vi "radius_plot.vi"(0 "Img Data In":T2, 11 "Controls In":T1) -> (2 "Integrated Intensity \n(Radias Direction)":i32[](graph), 4 "Img Data Out":T2, 15 "Controls Out":T1)   [LabVIEW 2023]
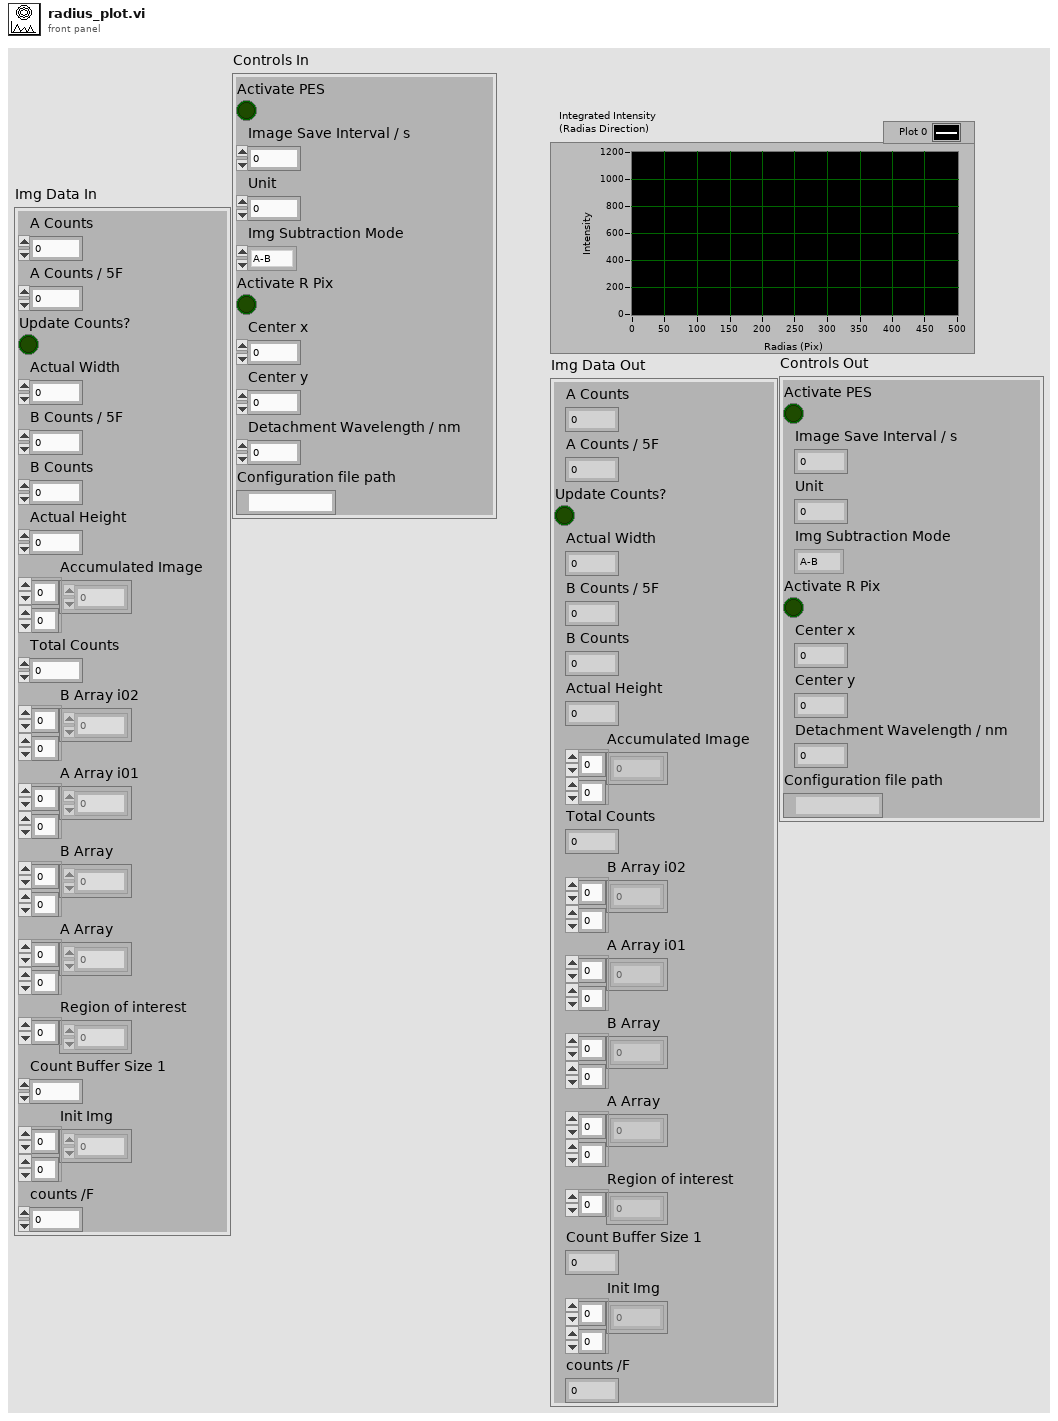
[diagram p1: front panel]
types:
  T1 = cluster{"Activate PES":bool, "Image Save Interval / s":dbl, "Unit":u16, "Img Subtraction Mode":enum16{"A-B", "B-A", "A+B"}, "Activate R Pix":bool, "Center x":i32, "Center y":i32, "Detachment Wavelength / nm":dbl, "Configuration file path":path}
  T2 = cluster{"A Counts":i32, "A Counts / 5F":dbl, "Update Counts?":bool, "Actual Width":u32, "B Counts / 5F ":dbl, "B Counts":i32, "Actual Height":u32, "Accumulated Image ":i16[][], "Total Counts":i32, "B Array i02":sgl[][], "A Array i01":sgl[][], "B Array":i16[][], "A Array":i16[][], "Region of interest":i32[], "Count Buffer Size 1":i32, "Init Img":i16[][], "counts /F":i16}
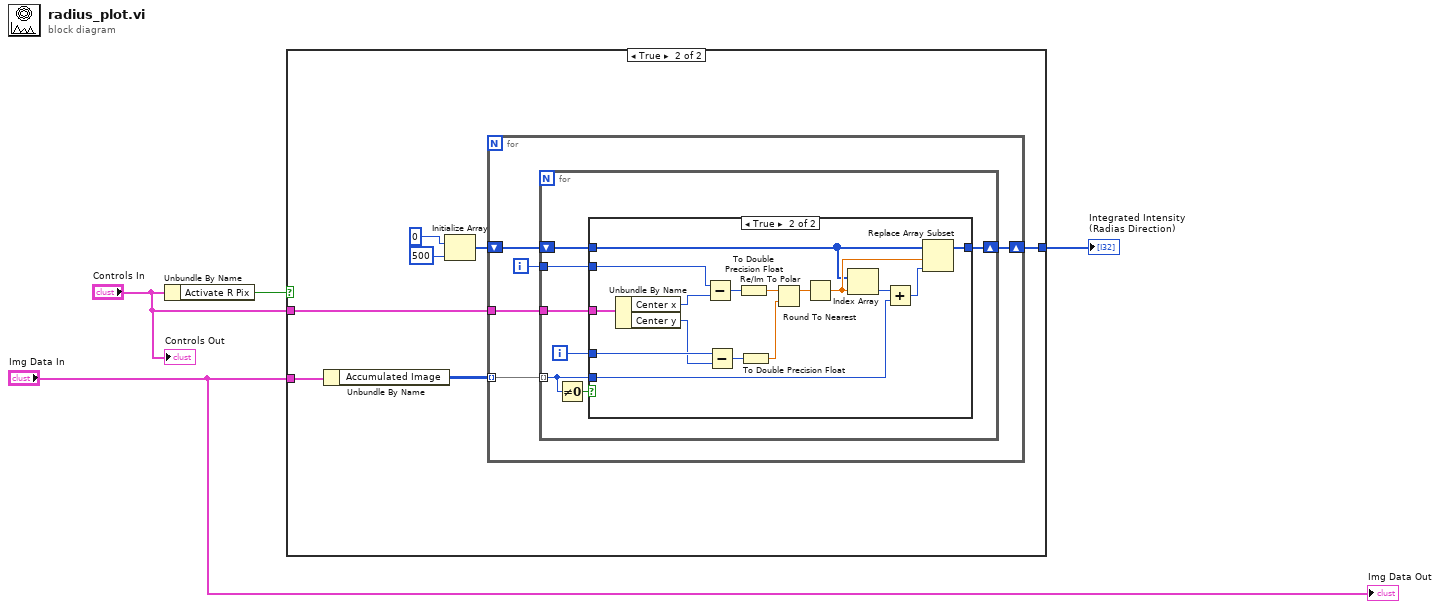
[diagram p0: block diagram]
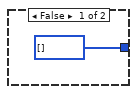
[diagram p2: hidden frame]
diagram:
  n1 = Unbundle By Name("Controls In") -> ("Activate R Pix"=w3:bool)
  n2 = case shown="True" w3 {
    tunnel: "Img Data In" -> [_ w9]
    tunnel: [i32[] [] w7] -> w2
    tunnel: "Controls In" -> [_ w6]
    frame False {
    }
    frame True {
      n3 = Unbundle By Name(w9) -> ("Accumulated Image"=w8:i16[][])
      n4 = Initialize Array(0, 500) -> (w12:i32[])
      n5 = for {
        tunnel: w8 -> [w17] mode=indexing
        shift-right: [w14] -> w7
        shift-left: w12 -> [w15]
        tunnel: w6 -> [w13]
        i -> [w16]
        n6 = for {
          tunnel: w17 -> [w21] mode=indexing
          tunnel: w16 -> [w22]
          shift-right: [w19] -> w14
          shift-left: w15 -> [w20]
          tunnel: w13 -> [w18]
          i -> [w23]
          n7 = Not Equal To 0?(x=w21) -> (x != 0?=w24:bool)
          n8 = case shown="True" w24 {
            tunnel: w23 -> [_ w36]
            tunnel: w22 -> [_ w35]
            tunnel: w21 -> [_ w34]
            tunnel: w20 -> [w25 w33]
            tunnel: [w25 w32] -> w19
            tunnel: w18 -> [_ w28]
            frame False {
            }
            frame True {
              n9 = Unbundle By Name(w28) -> ("Center x"=w27:i32, "Center y"=w26:i32)
              n10 = Subtract(x=w35, y=w27) -> (x-y=w37:i32)
              n11 = Subtract(x=w36, y=w26) -> (x-y=w38:i32)
              n12 = To Double Precision Float(number=w37) -> (double precision float=w31:dbl)
              n13 = To Double Precision Float(number=w38) -> (double precision float=w30:dbl)
              n14 = Re/Im To Polar(2:w30, 3:w31) -> (1:w29:dbl)  [unwired: 1 out]
              n15 = Round To Nearest(number=w29) -> (nearest integer value=w39:dbl)
              n16 = Index Array(array=w33, index=w39) -> (element=w41:i32)
              n17 = Add(x=w41, y=w34) -> (x+y=w40:i32)
              n18 = Replace Array Subset(array=w33, new element=w40, index=w39) -> (w32:i32[])
            }
          }
        }
      }
    }
  }
  "Integrated Intensity \n(Radias Direction)" <- w2
  "Img Data Out" <- "Img Data In"
  "Controls Out" <- "Controls In"
